vi "ImageCentroidCal c.vi"(10 "Clip Threshold":dbl, 11 "input array":u8[][](array[numeric])=array1024x1280[1310720 elements]) -> (0 "standard dev Col":dbl, 1 "standard dev Row":dbl, 2 "Centroid of Cols":dbl, 3 "Centroid of Rows":dbl, 4 "fitted center Col":dbl, 5 "min value":u8, 6 "fitted center Row":dbl, 7 "max value":u8, 8 "XY Graph":cluster{i32[], "Best Gaussian Fit":dbl[]}[](graph))   [LabVIEW 2013]
uses:
  <vilib>/Analysis/6fits.llb/Curve Fitting Criteria.ctl
  <vilib>/Analysis/NI_AALPro.lvlib
panel:
  out "Video":u8[][](graph)
  out "Best Gaussian Fit Col":dbl[](array[numeric])
  out "offset Col":dbl=1.0
  out "amplitude Col":dbl
  in  "initial guess Cols":T1={"initial amplitude"=1000.0, "initial center"=500.0, "initial standard deviation"=10.0, "offset"=1.0}
  out "Best Gaussian Fit Row":dbl[](array[numeric])
  out "offset Row":dbl=1.0
  out "amplitude Row":dbl
  in  "parameter bounds":T2={"amp min"=0.0, "amp max"=4000.0, "center min"=0.0, "center max"=1200.0, "dev min"=1.0, "dev max"=500.0, "offset min"=0.0, "offset max"=1000.0}
  in  "initial guess Rows":T1={"initial amplitude"=1000.0, "initial center"=500.0, "initial standard deviation"=10.0, "offset"=1.0}
  out "min index(es)":i32[](array[numeric])
  out "max index(es)":i32[](array[numeric])
  out "input array size row, col":i32[](array[numeric])
  # "2 sigma = 1/e^2 (13.5%) radius\nFWHM = 2.35 sigma"
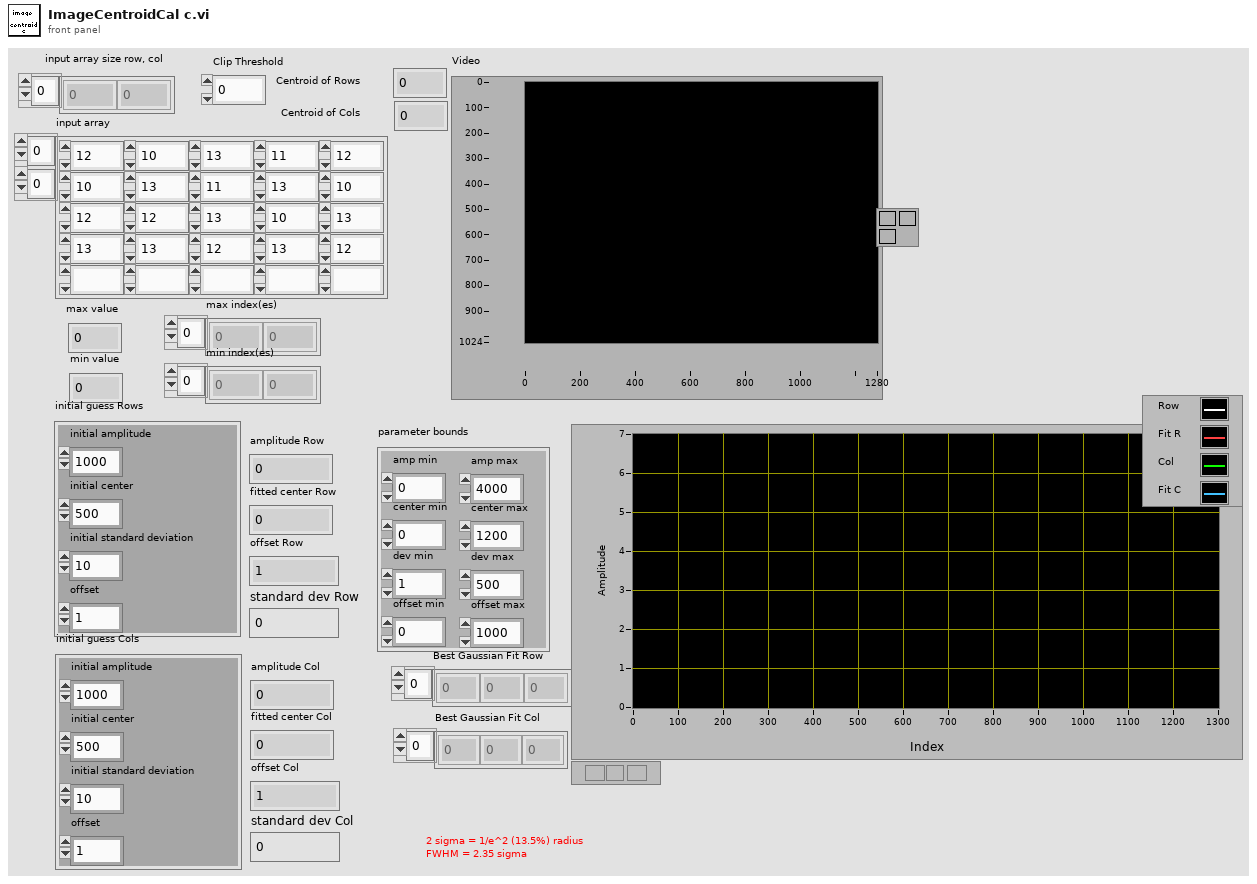
[diagram p1: front panel]
types:
  T1 = cluster{"initial amplitude":dbl, "initial center":dbl, "initial standard deviation":dbl, "offset":dbl}
  T2 = cluster{"amp min":dbl, "amp max":dbl, "center min":dbl, "center max":dbl, "dev min":dbl, "dev max":dbl, "offset min":dbl, "offset max":dbl}
  T3 = typedef "NI_AALPro.lvlib/Curve Fitting Criteria.ctl" = u16
  T4 = cluster{"Index Array":i32[], "Best Gaussian Fit":dbl[]}
  T5 = cluster{"Index Array":i32[], "Best Gaussian Fit":dbl[]}[]
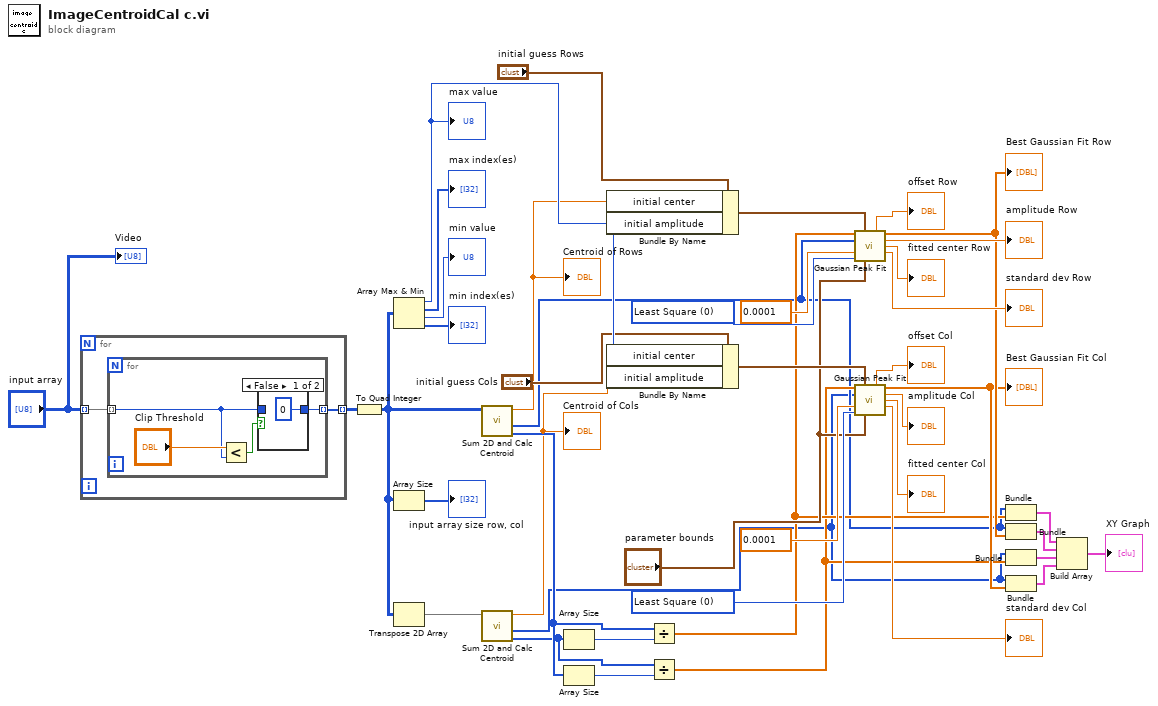
[diagram p0: block diagram]
diagram:
  w27 = T3 0 items=["Least Square", "Least Absolute Residual", "Bisquare"] ("method")
  w39 = T3 0 items=["Least Square", "Least Absolute Residual", "Bisquare"] ("method")
  n1 = for {
    tunnel: "input array" -> [w45] mode=indexing
    tunnel: [w44] -> w10 mode=indexing
    n2 = for {
      tunnel: w45 -> [w48] mode=indexing
      tunnel: [w46] -> w44 mode=indexing
      n3 = Less?(x="Clip Threshold", y=w48) -> (x < y?=w47:bool)
      n4 = case shown="False" w47 {
        tunnel: w48 -> [_ w51]
        tunnel: [0 w51] -> w46
        frame False {
        }
        frame True {
        }
      }
    }
  }
  n5 = To Quad Integer(1:w10) -> (0:w9:i64[][])
  n6 = Array Max & Min(array=w9) -> (max value=w19:i64, max index (indices)=→"max index(es)":i32[], min value=→"min value":i64, min index (indices)=→"min index(es)":i32[])
  "max value" <- w19
  n7 = Array Size(array=w9) -> (size(s)=→"input array size row, col":i32[])
  n8 = Transpose 2D Array(2D array=w9) -> (transposed array=w5:i64[][])
  n9 = call "Sum 2D and Calc Centroid.vi"("input array"=w9) -> ("Summed Array"=w6:i64[], "Index Array"=w7:i32[], "Centroid"=w8:dbl)  [unwired: 8 in]
  "Centroid of Rows" <- w8
  n10 = call "Sum 2D and Calc Centroid.vi"("input array"=w5) -> ("Summed Array"=w3:i64[], "Index Array"=w2:i32[], "Centroid"=w4:dbl)  [unwired: 8 in]
  "Centroid of Cols" <- w4
  n11 = Array Size(array=w3) -> (size(s)=w14:i32)
  n12 = Array Size(array=w6) -> (size(s)=w12:i32)
  n13 = Bundle By Name(cluster="initial guess Rows", "initial center"=w8, "initial amplitude"=w19) -> (w29:T1)
  n14 = Bundle By Name(cluster="initial guess Cols", "initial center"=w4, "initial amplitude"=w19) -> (w21:T1)
  n15 = Divide(x=w6, y=w14) -> (x/y=w13:dbl[])
  n16 = Divide(x=w3, y=w12) -> (x/y=w11:dbl[])
  n17 = call <vilib>:"Gaussian Peak Fit.vi"("Y"=w13, "initial guess"=w29, "X"=w7, "tolerance"=0.0001, "method"=w39, "parameter bounds"="parameter bounds") -> ("offset"=→"offset Row":dbl, "Best Gaussian Fit"=w34:dbl[], "amplitude"=→"amplitude Row":dbl, "center"=→"fitted center Row":dbl, "standard deviation"=→"standard dev Row":dbl)  [unwired: 3 in, 2 out]
  "Best Gaussian Fit Row" <- w34
  n18 = call <vilib>:"Gaussian Peak Fit.vi"("Y"=w11, "initial guess"=w21, "X"=w2, "tolerance"=0.0001, "method"=w27, "parameter bounds"="parameter bounds") -> ("offset"=→"offset Col":dbl, "Best Gaussian Fit"=w22:dbl[], "amplitude"=→"amplitude Col":dbl, "center"=→"fitted center Col":dbl, "standard deviation"=→"standard dev Col":dbl)  [unwired: 3 in, 2 out]
  "Best Gaussian Fit Col" <- w22
  n19 = Bundle("Index Array"=w7, w13) -> (w33:cluster{"Index Array":i32[], dbl[]})  [unwired: 1 in]
  n20 = Bundle("Index Array"=w7, "Best Gaussian Fit"=w34) -> (w32:T4)  [unwired: 1 in]
  n21 = Bundle("Index Array"=w2, w11) -> (w18:cluster{"Index Array":i32[], dbl[]})  [unwired: 1 in]
  n22 = Bundle("Index Array"=w2, "Best Gaussian Fit"=w22) -> (w17:T4)  [unwired: 1 in]
  n23 = Build Array(w33, w32, w18, w17) -> (→"XY Graph":T5)
  "Video" <- "input array"
